vi "Click Position.vi"(7 "XY Graph Ref":refnum<vi>, 8 "error in":errorcluster, 11 "Click Coords":T2) -> (0 "error out":errorcluster, 3 "Operation":T1(ring))   [LabVIEW 2015, in "Teaching View.lvlib" / "Teaching View XControl.xctl"]
doc: "Determines the area in which the operator is mousing in. This will determine the mouse cursor to use"
uses:
  Teaching View XControl.xctl
  <vilib>/Utility/miscctls.llb/LVPoint32TypeDef.ctl
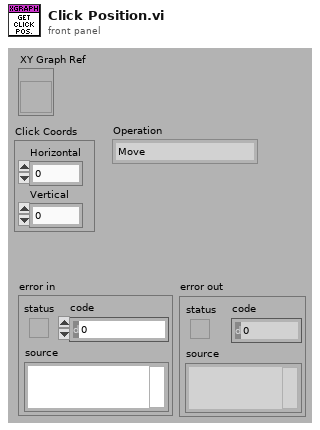
[diagram p1: front panel]
types:
  T1 = enum16{"Move", "left cursor", "right cursor", "none"}
  T2 = typedef "LVPoint32TypeDef.ctl" = cluster{"Horizontal":i32, "Vertical":i32}
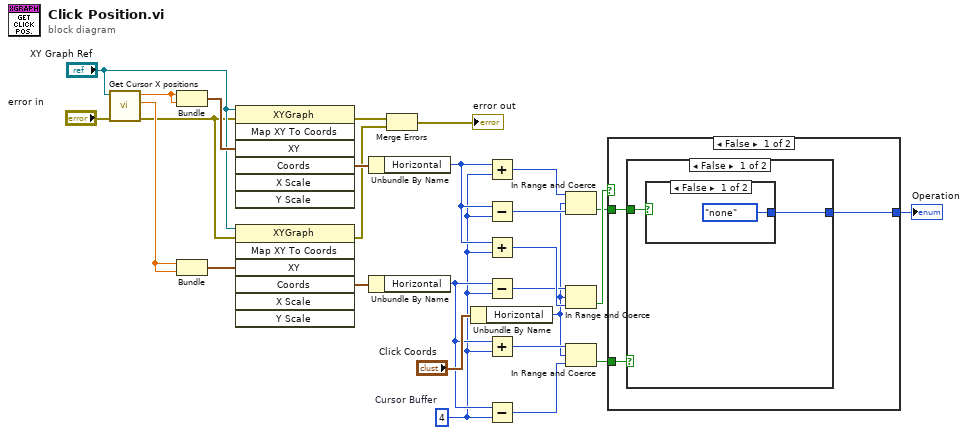
[diagram p0: block diagram]
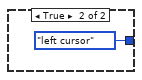
[diagram p2: hidden frame]
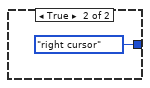
[diagram p3: hidden frame]
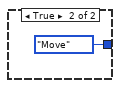
[diagram p4: hidden frame]
diagram:
  w8 = 4  # Cursor Buffer
  n1 = call "Get Cursor X positions.vi"("error in"="error in", "XY Graph Ref"="XY Graph Ref") -> ("error out"=w4:errorcluster, "Right"=w22:dbl, "Left"=w21:dbl)  [unwired: 6 in, 1 out]
  n2 = Bundle("Left"=w21, "Left"=w21) -> (w23:cluster{"Left":dbl, "Left":dbl})  [unwired: 1 in]
  n3 = Bundle("Right"=w22, "Right"=w22) -> (w27:cluster{"Right":dbl, "Right":dbl})  [unwired: 1 in]
  n4 = invoke on="Invoke Node" class="XYGraph" method="Map XY To Coords"(reference="XY Graph Ref", error in=w4, "XY"=w23) -> (error out=w2:errorcluster, "Coords"=w24:T2)  [unwired: 4 in, 5 out]
  n5 = invoke on="Invoke Node" class="XYGraph" method="Map XY To Coords"(reference="XY Graph Ref", error in=w4, "XY"=w27) -> (error out=w1:errorcluster, "Coords"=w26:T2)  [unwired: 4 in, 5 out]
  n6 = Unbundle By Name(w24) -> ("Horizontal"=w9:i32)
  n7 = Unbundle By Name(w26) -> ("Horizontal"=w15:i32)
  n8 = Merge Errors(w2, w1) -> (→"error out":errorcluster)
  n9 = Unbundle By Name("Click Coords") -> ("Horizontal"=w7:i32)
  n10 = Add(x=w9, y=w8) -> (x+y=w10:i32)
  n11 = Subtract(x=w9, y=w8) -> (x-y=w11:i32)
  n12 = Add(x=w9, y=w8) -> (x+y=w19:i32)
  n13 = Subtract(x=w15, y=w8) -> (x-y=w18:i32)
  n14 = Add(x=w15, y=w8) -> (x+y=w14:i32)
  n15 = Subtract(x=w15, y=w8) -> (x-y=w13:i32)
  n16 = In Range and Coerce(upper limit=w10, x=w7, lower limit=w11) -> (In Range?=w6:bool)  [unwired: 1 out]
  n17 = In Range and Coerce(upper limit=w18, x=w7, lower limit=w19) -> (In Range?=w17:bool)  [unwired: 1 out]
  n18 = In Range and Coerce(upper limit=w14, x=w7, lower limit=w13) -> (In Range?=w12:bool)  [unwired: 1 out]
  n19 = case shown="False" w17 {
    tunnel: [w30 T1."Move" ("Operation")] -> w16
    tunnel: w12 -> [w29 _]
    tunnel: w6 -> [w28 _]
    frame False {
      n20 = case shown="False" w29 {
        tunnel: [w32 T1."right cursor" ("Operation")] -> w30
        tunnel: w28 -> [w31 _]
        frame False {
          n21 = case shown="False" w31 {
            tunnel: [T1."none" ("Operation") T1."left cursor" ("Operation")] -> w32
            frame False {
            }
            frame True {
            }
          }
        }
        frame True {
        }
      }
    }
    frame True {
    }
  }
  "Operation" <- w16
